vi "Start UI.vi"() -> ()   [LabVIEW 2026, in "App Controller.lvclass"]
uses:
  App Controller.lvclass
  App Controller.lvclass/App Controller.ctl
  UI/Shell UI/Shell UI.lvclass
panel:
  in  "App Controller in":refnum<class "App Controller.lvclass">
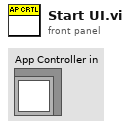
[diagram p1: front panel]
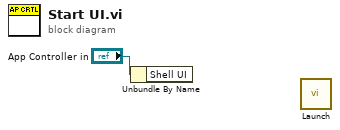
[diagram p0: block diagram]
diagram:
  n1 = Unbundle By Name("App Controller in") -> ()  [unwired: 1 out]
  n2 = call "Launch.vi"() -> ()  [unwired: 12 in]
